vi "Add Handler(by Ref).vi"(8 "error in (no error)":errorcluster, 10 "Handler":refnum<class "Handler.lvclass">) -> (0 "error out":errorcluster)   [LabVIEW 2017, in "Error Log.lvlib" / "Logger.lvclass"]
doc: "Adds the <b>Handler</b> to the referenced Logger."
uses:
  Logger.lvclass
  Handler/Handler.lvclass
  Logger.lvclass/Logger.ctl
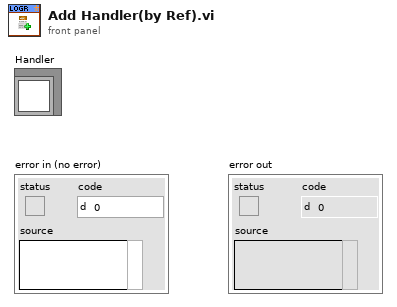
[diagram p1: front panel]
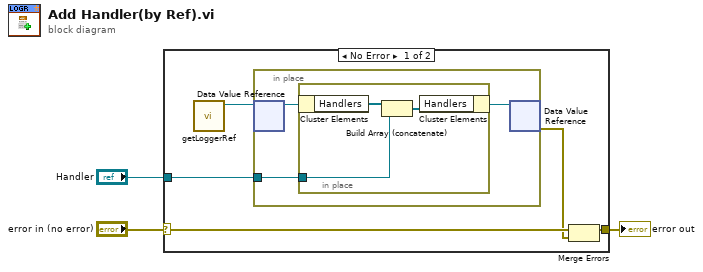
[diagram p0: block diagram]
diagram:
  n1 = case shown="No Error" "error in (no error)" {
    selector: "error in (no error)" -> [w8 w15]
    tunnel: [w6 w15] -> w3
    tunnel: "Handler" -> [w7 _]
    frame No Error {
      n2 = call "getLoggerRef.vi"() -> ("Logger Ref"=w4:refnum<data-value>)  [unwired: 10 in, 1 out]
      n3 = in-place {
        in-place-border: w7 -> [w11]
        n4 = in-place-dvr #1(w4) -> (w10:refnum<class "Logger.lvclass">)  [unwired: 1 out]
        n5 = in-place {
          in-place-border: w11 -> [w14]
          n6 = in-place-cluster #2(w10) -> ("Handlers"=w13:refnum<class "Handler.lvclass">[])
          n7 = Build Array (concatenate)(w13, w14) -> (w12:refnum<class "Handler.lvclass">[])
          n8 = in-place-cluster #2("Handlers"=w12) -> (w9:refnum<class "Logger.lvclass">)
        }
        n9 = in-place-dvr #1(w9) -> (w5:errorcluster)  [unwired: 1 out]
      }
      n10 = Merge Errors(w8, w5) -> (w6:errorcluster)
    }
    frame Error {
    }
  }
  "error out" <- w3
